vi "MAC DEL.vi"(0 "System no.":i32=1 min=1 max=4 step=1, 2 "Macro name":string, 3 "With dialog?":bool=TRUE, 5 "error in":errorcluster) -> (14 "Controller error":bool, 19 "error out":errorcluster)   [LabVIEW 2020]
doc: "Delete macro. If \"With dialog\" is TRUE, a dialog box pops up to confirm the deletion. \"Controller error\" is TRUE if selected system reports an error code which is not zero.\n\nE-516: Changes not saved with WPA.vi are only present in RAM and will be lost when the controller is powered off.\n\nE-816: Changes not saved with WPA.vi are only present in RAM and will be lost when the controller is powered off. This command cannot be issued to a slave. Check controller manual to find out if MAC BEG is supported.\n\nM-8X0: Only for GCS syntax version = GCS 2.0 or higher (check with CSV?.vi. If CSV?.vi is not supported, syntax version is GCS 1.0)."
panel:
  # "Delete macro. If \"With dialog\" is TRUE, a dialog box pops\nup to confirm the deletion."
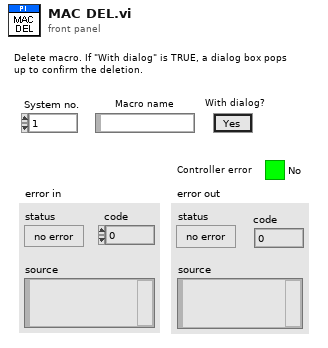
[diagram p1: front panel]
types:
  T1 = enum16{"Disable error check", "Force error check", "Use global settings"}
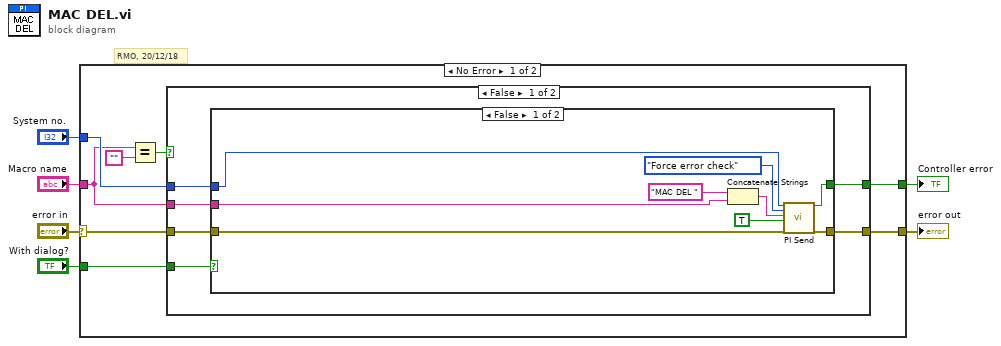
[diagram p0: block diagram]
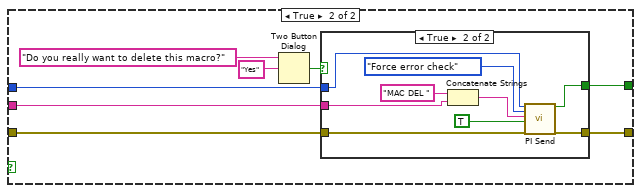
[diagram p2: hidden frame]
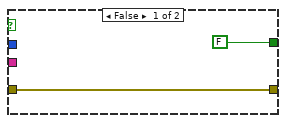
[diagram p3: hidden frame]
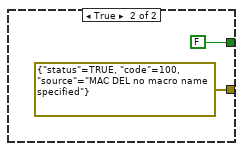
[diagram p4: hidden frame]
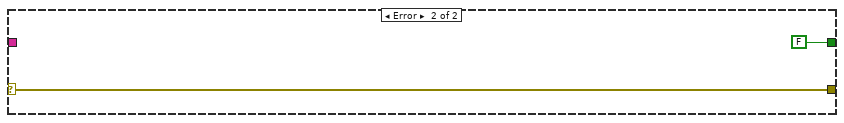
[diagram p5: hidden frame]
diagram:
  # "RMO, 20/12/18"
  n1 = case shown="No Error" "error in" {
    selector: "error in" -> [w7 w51]
    tunnel: [w14 w51] -> w6
    tunnel: "System no." -> [w13 _]
    tunnel: [w12 FALSE ("Controller error")] -> w4
    tunnel: "With dialog?" -> [w11 _]
    tunnel: "Macro name" -> [w9 _]
    frame No Error {
      n2 = Equal?(x=w9, y="") -> (x = y?=w8:bool)
      n3 = case shown="False" w8 {
        tunnel: w7 -> [w20 _]
        tunnel: [w19 errorcluster {"status"=TRUE, "code"=100, "source"="MAC DEL no macro name specified"} ("error out")] -> w14
        tunnel: w13 -> [w18 _]
        tunnel: [w17 FALSE] -> w12
        tunnel: w11 -> [w16 _]
        tunnel: w9 -> [w15 _]
        frame False {
          n4 = case shown="False" w16 {
            tunnel: w20 -> [w29 w37]
            tunnel: [w23 w36] -> w19
            tunnel: w18 -> [w26 w35]
            tunnel: [w22 w34] -> w17
            tunnel: w15 -> [w24 w33]
            frame False {
              n5 = Concatenate Strings("MAC DEL ", w24) -> (w25:string)
              n6 = call "PI Send.vi"("System no."=w26, "Error check settings"=T1."Force error check", "String to send"=w25, "Attach termination char.?"=TRUE ("Attach Linefeed?"), "error in"=w29) -> ("Controller error"=w22:bool, "error out"=w23:errorcluster)  [unwired: 1 in, 12 out]
            }
            frame True {
              n7 = Two Button Dialog(message="Do you really want to delete this macro?", 2:"Yes" ("T button name (\"OK\")")) -> (T button?=w30:bool)  [unwired: 1 out]
              n8 = case shown="True" w30 {
                tunnel: w37 -> [w38 w48]
                tunnel: [w38 w42] -> w36
                tunnel: w35 -> [_ w45]
                tunnel: [FALSE w41] -> w34
                tunnel: w33 -> [_ w43]
                frame False {
                }
                frame True {
                  n9 = Concatenate Strings("MAC DEL ", w43) -> (w44:string)
                  n10 = call "PI Send.vi"("System no."=w45, "Error check settings"=T1."Force error check", "String to send"=w44, "Attach termination char.?"=TRUE ("Attach Linefeed?"), "error in"=w48) -> ("Controller error"=w41:bool, "error out"=w42:errorcluster)  [unwired: 1 in, 12 out]
                }
              }
            }
          }
        }
        frame True {
        }
      }
    }
    frame Error {
    }
  }
  "error out" <- w6
  "Controller error" <- w4
